vi "Write Condition.vi"(8 "error in (no error)":errorcluster, 9 "Samples":refnum<class "Sample.lvclass">[](array[class]), 10 "Action (Allow)":T1, 11 "Interlock Sample in":refnum<class "Interlock Sample.lvclass">) -> (0 "error out":errorcluster, 3 "Interlock Sample out":refnum<class "Interlock Sample.lvclass">)   [LabVIEW 2015, in "cRIO-Carbondioxide.lvlib" / "Interlock Sample.lvclass"]
uses:
  Interlock Sample.lvclass
  subs/Sample/Sample.lvclass
  Action Enum.ctl
  Interlock Sample.lvclass/Interlock Sample.ctl
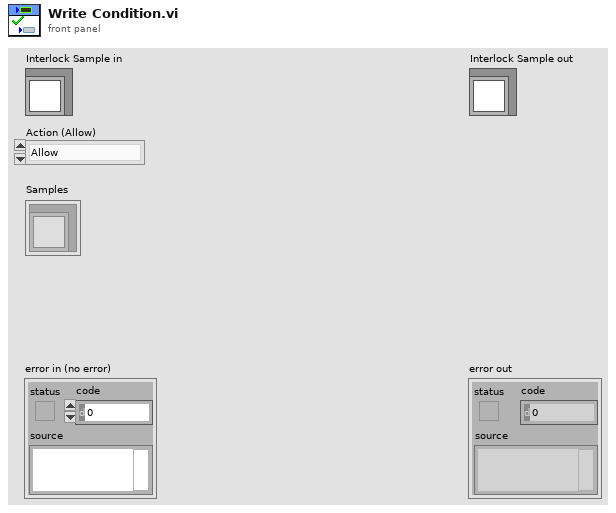
[diagram p1: front panel]
types:
  T1 = typedef "Action Enum.ctl" = enum16{"Allow", "Deny"}
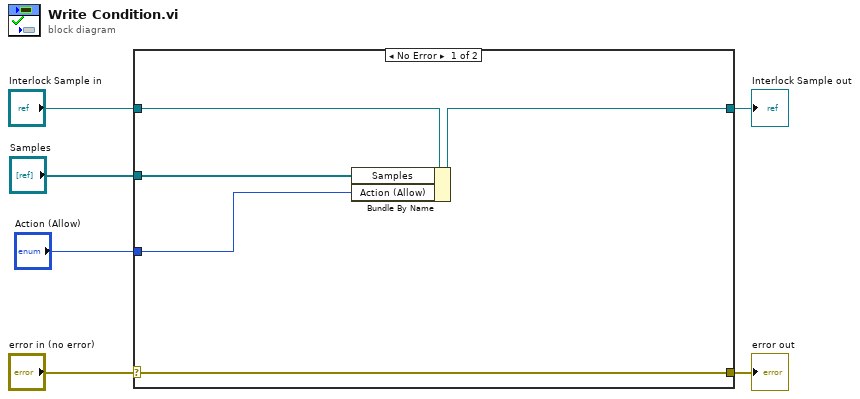
[diagram p0: block diagram]
diagram:
  n1 = case shown="No Error" "error in (no error)" {
    selector: "error in (no error)" -> [w10 w13]
    tunnel: [w10 w13] -> w5
    tunnel: [w9 w12] -> w3
    tunnel: "Interlock Sample in" -> [w11 w12]
    tunnel: "Samples" -> [w8 _]
    tunnel: "Action (Allow)" -> [w7 _]
    frame No Error {
      n2 = Bundle By Name(cluster=w11, "Samples"=w8, "Action (Allow)"=w7) -> (w9:refnum<class "Interlock Sample.lvclass">)
    }
    frame Error {
    }
  }
  "error out" <- w5
  "Interlock Sample out" <- w3
